vi "Write Handle.vi"(8 "error in (no error)":errorcluster, 10 "NI DMM":refnum<k15>, 11 "NI DMM Driver in":refnum<class "DMM.NI.lvclass">) -> (0 "error out":errorcluster, 3 "NI DMM Driver out":refnum<class "DMM.NI.lvclass">)   [LabVIEW 2020, in "NI DMM Driver.lvlib" / "DMM.NI.lvclass"]
doc: "Write the NI DMM Handle to the NI DMM Driver."
uses:
  DMM.NI.lvclass
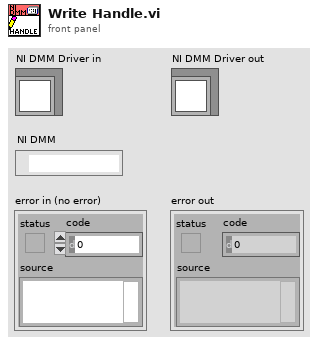
[diagram p1: front panel]
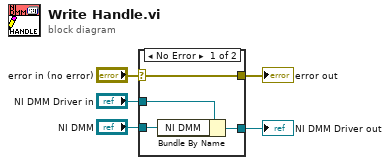
[diagram p0: block diagram]
diagram:
  n1 = case shown="No Error" "error in (no error)" {
    selector: "error in (no error)" -> [w9 w10]
    tunnel: [w9 w10] -> w4
    tunnel: [w7 w11] -> w2
    tunnel: "NI DMM Driver in" -> [w8 w11]
    tunnel: "NI DMM" -> [w6 _]
    frame No Error {
      n2 = Bundle By Name(cluster=w8, "NI DMM"=w6) -> (w7:refnum<class "DMM.NI.lvclass">)
    }
    frame Error {
    }
  }
  "error out" <- w4
  "NI DMM Driver out" <- w2
